vi "tefejaso def3.vi"() -> ()   [LabVIEW 2011]
panel:
  in  "show event/index":bool
  in  "Timeout UDP READ  ms":i32=548
  out "Receive Buffer Size":u32=548
  in  "activetimeout":bool
  out "Active Time Out":bool
  out "Buffer size":u32=548
  in  "Change UDP Parameters":bool
  out "Event Hex":string
  in  "show udp index":bool
  in  "see supertime sec":bool
  in  "see supertime  ns":bool
  in  "see channel":bool
  in  "see tot":bool
  in  "Show channel table":bool
  out "Num Pack 2":u32=1
  out "Supertime ns":u32=1
  out "Supertime sec":u32=1
  out "error time order":bool
  out "error channel":bool
  out "Num Pack":u32=1
  out "Veces canal":u32[](array[numeric])
  out "Table":string[][](table)
  out "num canal":i32=548
  out "Canal TDC":u32[](array[numeric])
  in  "desviacion tipica ancho":dbl
  in  "suma desviacon":dbl
  out "media pulso":dbl
  in  "suma ancho pulso":u32=1
  out "iteracion":i32
  in  "stop":bool
  out "error timestamp":bool
  out "ToT":dynamicdata(graph) caption="Histogram"
  out "Events/TDC channel":dynamicdata(graph) caption="Histogram"
  out "ToT":u32=1
  out "Arrival Time":u32=1
  out "Channel TDC":u32=1
  out "bufferfull":timestamp
  out "UDP INDEX":dynamicdata(graph) caption="Histogram"
  out "EVENT/index":dynamicdata(graph) caption="Histogram"
  out "indice":u32=1
  out "Supertime sec":dynamicdata(graph)
  out "supertime ns":dynamicdata(graph)
  out "current_HRV":u32=1
  out "current_fifo_afull":u32=1
  out "FIFO_FULL":bool[](array[boolean])
  out "HRV":bool[](array[boolean])
  out "Size Packet Bytes":i32
  out "Data Received":string
  in  "max bytes/read":i32=548
  in  "index":u32=1
  out "Port":u16=61557
  out "Num Event":u32=1
  out "START TIME":timestamp
  out "hold_fifo_afull":u32=1
  out "hold_HRV":u32=1
  in  "event/ts":u32=1
  in  "pak_loss":u32=1 caption="packet losses"
  in  "TS_Ch_1":u32=1
  in  "TS_Ch 2":u32=1
  in  "TS_Ch 3":u32=1
  in  "TS_Ch 4":u32=1
  in  "TS_Ch 5":u32=1
  in  "TS_Ch 6":u32=1
  in  "TS_Ch 7":u32=1
  in  "TS_Ch 8":u32=1
  in  "TS_Ch 9":u32=1
  in  "TS_Ch 10":u32=1
  in  "TS_Ch_0":u32=1
  in  "TS_Ch_13":u32=1
  in  "TS_Ch 12":u32=1
  in  "TS_Ch_14":u32=1
  in  "TS_Ch_11":u32=1
  in  "TS_Ch_15":u32=1
  in  "TS_Ch_16":u32=1
  in  "TS_Ch_18":u32=1
  in  "TS_Ch 19":u32=1
  in  "TS_Ch_20":u32=1
  in  "TS_Ch_17":u32=1
  in  "TS_Ch_21":u32=1
  in  "TS_Ch_22":u32=1
  in  "TS_Ch_24":u32=1
  in  "TS_Ch 25":u32=1
  in  "TS_Ch_26":u32=1
  in  "TS_Ch_23":u32=1
  in  "TS_Ch_27":u32=1
  in  "TS_Ch_28":u32=1
  in  "TS_Ch_29":u32=1
  in  "TS_Ch_30":u32=1
  # "TDC DATA MONITOR"
  # "UDP TRANSFER CONDITIONS"
  # "TRANSFER ERRORS"
  # "PACKET INFORMATION"
  # "EVENT INFORMATION"
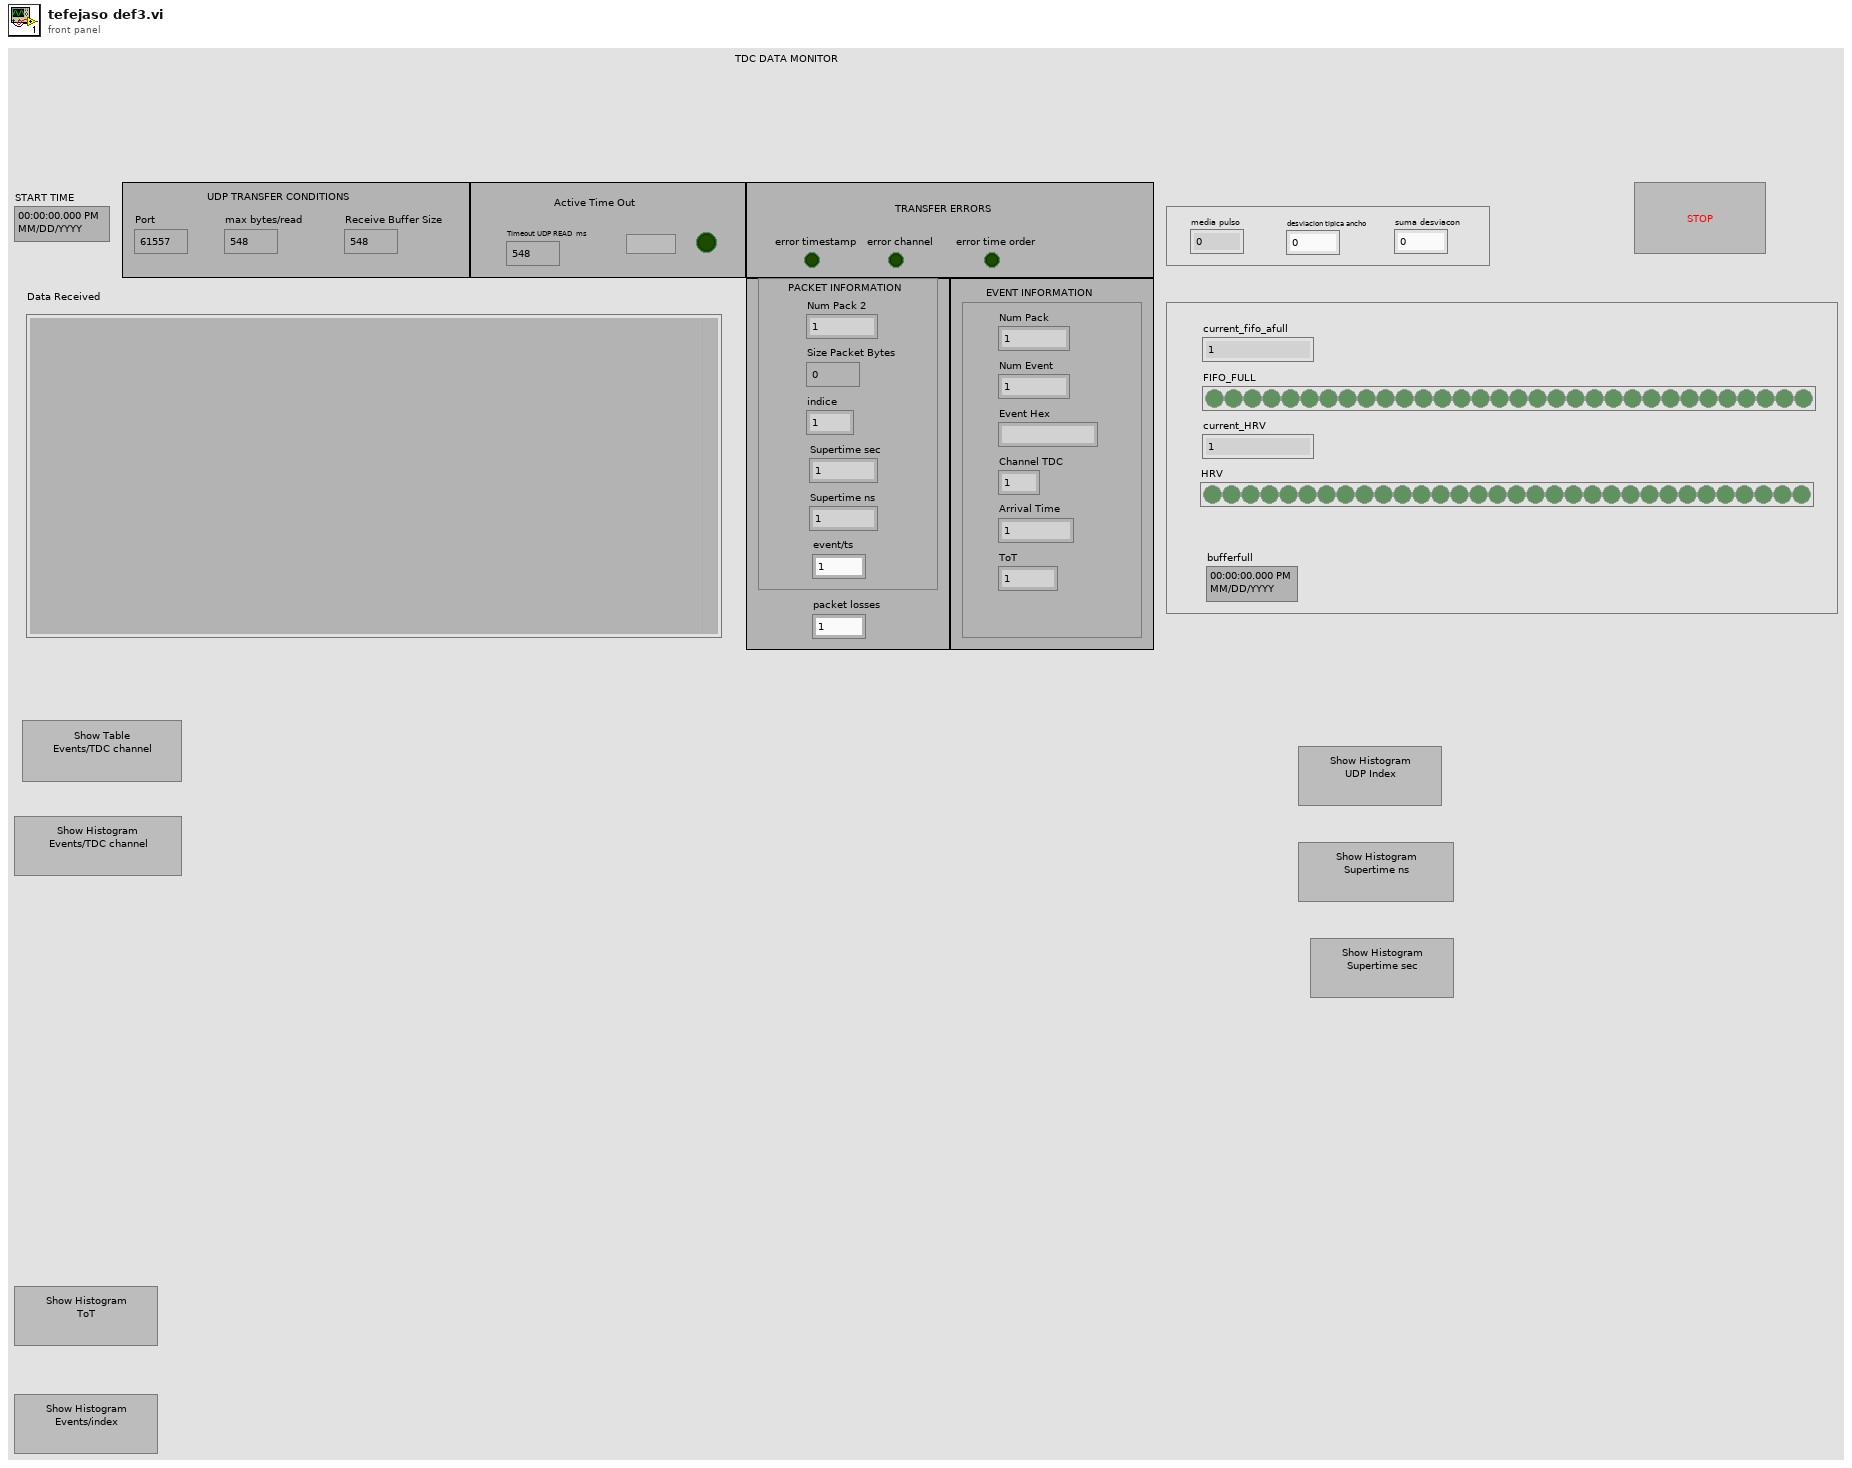
[diagram p1: front panel]
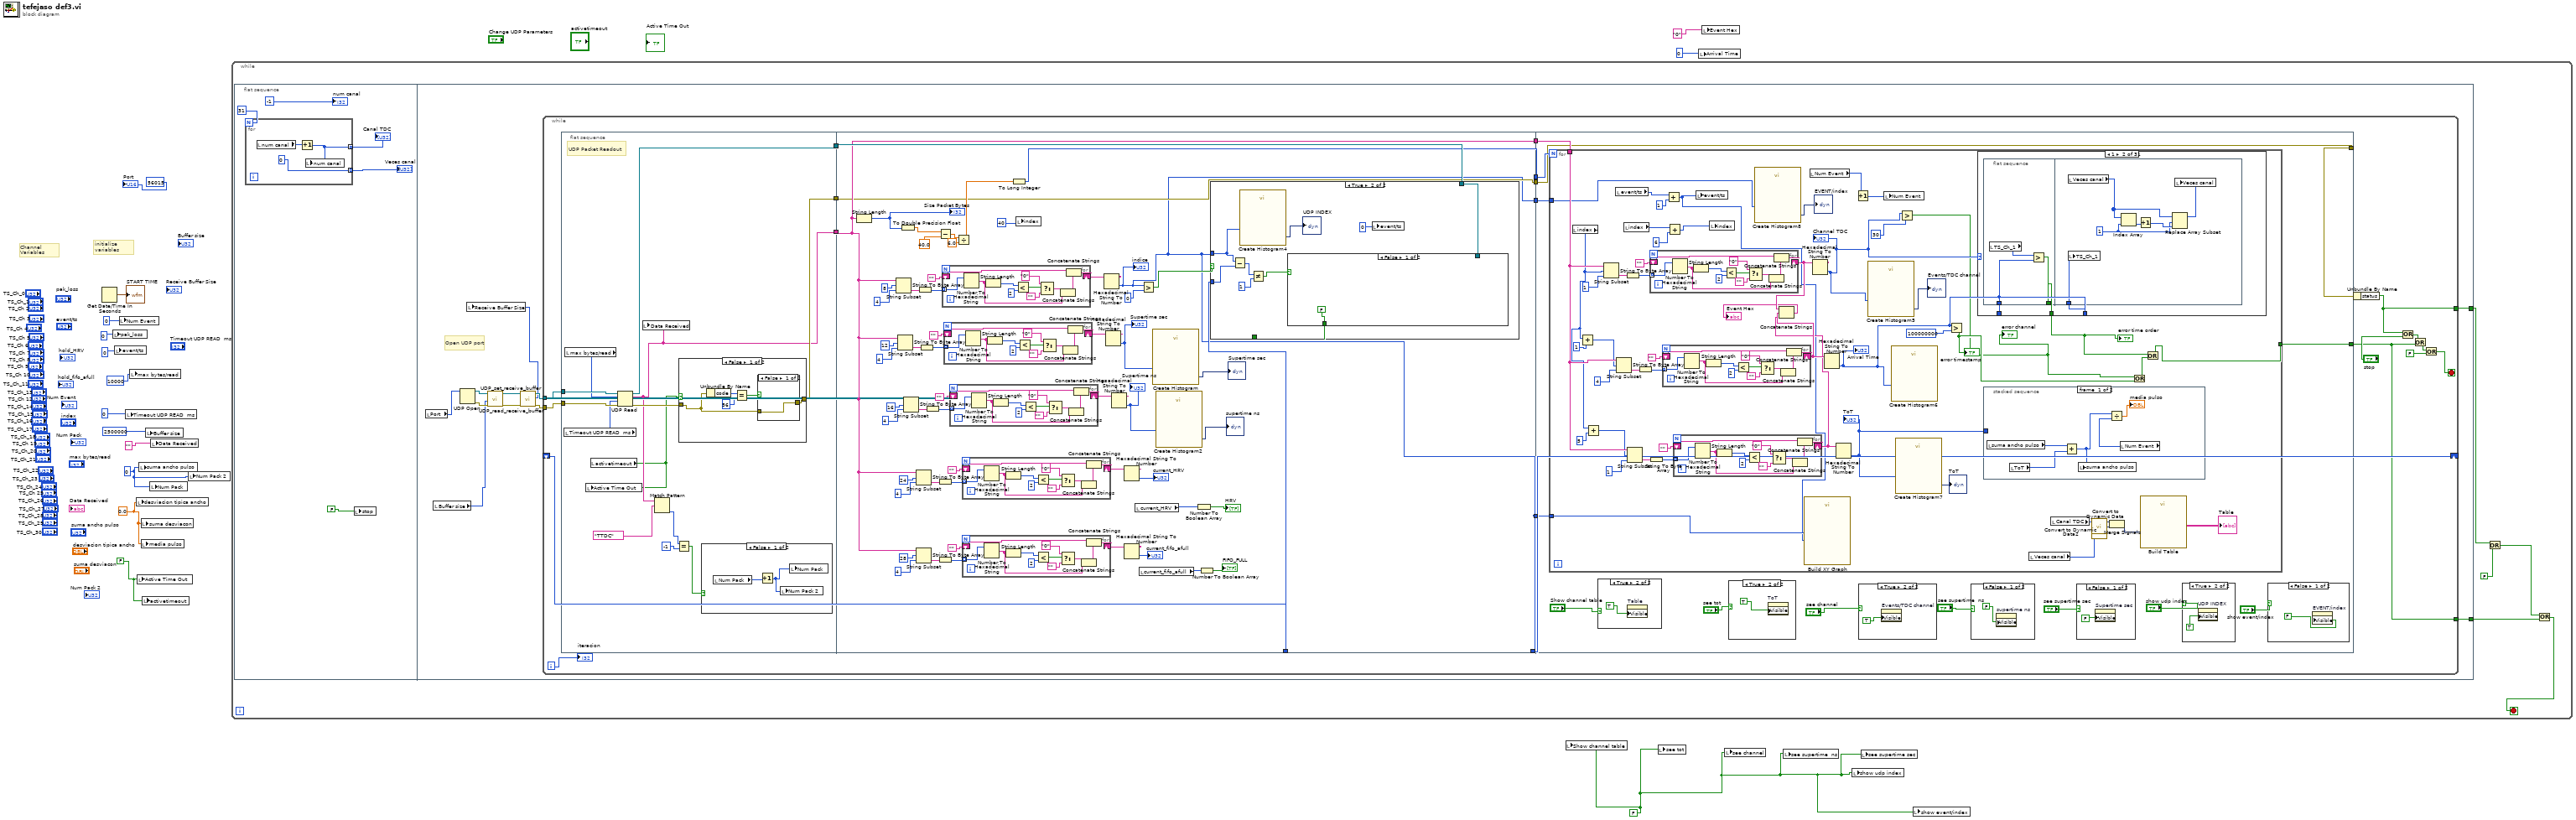
[diagram p0: block diagram]
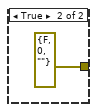
[diagram p2: hidden frame]
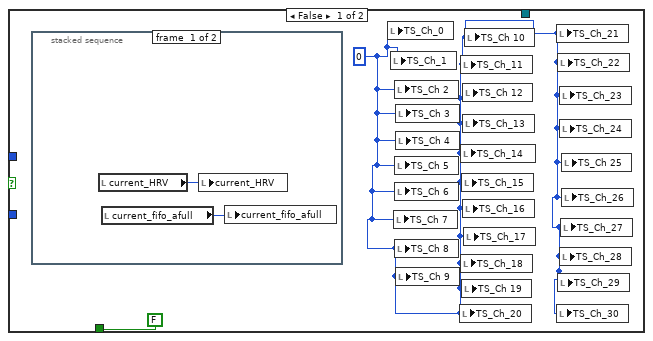
[diagram p5: hidden frame]
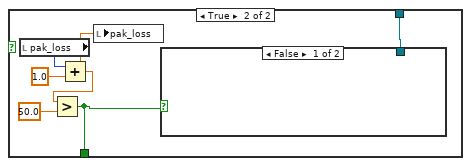
[diagram p7: hidden frame]
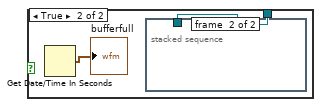
[diagram p8: hidden frame]
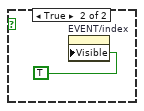
[diagram p10: hidden frame]
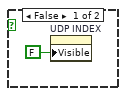
[diagram p11: hidden frame]
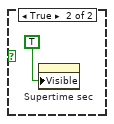
[diagram p12: hidden frame]
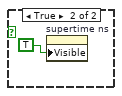
[diagram p13: hidden frame]
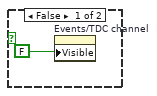
[diagram p14: hidden frame]
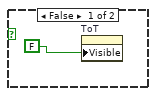
[diagram p15: hidden frame]
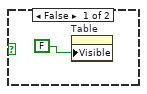
[diagram p16: hidden frame]
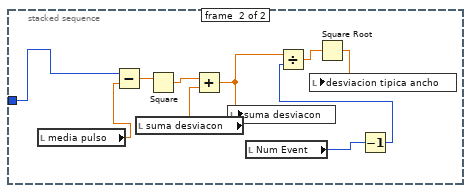
[diagram p17: hidden frame]
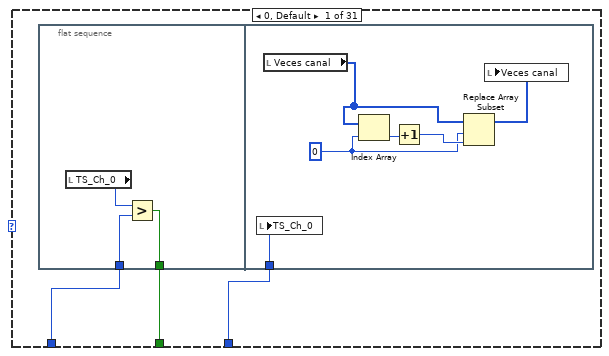
[diagram p18: hidden frame]
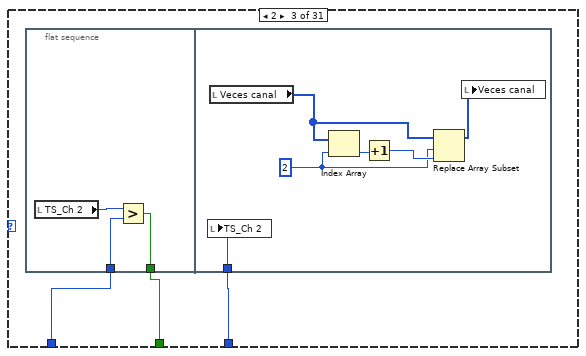
[diagram p19: hidden frame]
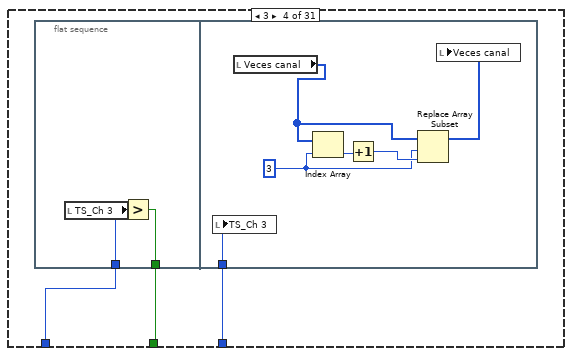
[diagram p20: hidden frame]
diagram:
  w1 = FALSE
  w5 = FALSE
  w9 = 0.0
  w8 = u32 0 ("event/ts")
  # "initialize variables"
  # "Channel Variables"
  n1 = Get Date/Time In Seconds() -> (seconds since 1Jan1904=→"START TIME":timestamp)
  n2 = local write "pak_loss"(u32 0 ("pak_loss")) -> ()
  n3 = local write "event/ts"(u32 0 ("event/ts")) -> ()
  n4 = local write "Num Event"(u32 0 ("contador eventos")) -> ()
  n5 = local write "Timeout UDP READ  ms"(0 ("event/ts")) -> ()
  n6 = local write "max bytes/read"(10000) -> ()
  n7 = local write "desviacion tipica ancho"(w9) -> ()
  n8 = local write "Active Time Out"(w5) -> ()
  n9 = local write "suma ancho pulso"(w8) -> ()
  n10 = local write "suma desviacon"(w9) -> ()
  n11 = local write "media pulso"(w9) -> ()
  n12 = local write "activetimeout"(w5) -> ()
  n13 = local write "Buffer size"(u32 2500000 ("Receive Buffer Size")) -> ()
  n14 = local write "Num Pack"(w8) -> ()
  n15 = local write "Data Received"("") -> ()
  n16 = local write "Num Pack 2"(w8) -> ()
  n17 = while {
    stop <- w17 stop-if-true
    n18 = flat-sequence {
      tunnel: [w33] -> w20
      tunnel: [w29] -> w18
      frame #0 {
        n19 = for {
          N: 31 ("contador eventos") -> [_]
          tunnel: [w27] -> w24 mode=indexing
          tunnel: [u32 0 ("contador eventos")] -> w25 mode=indexing
          n20 = local read "num canal"() -> (w28:i32)
          n21 = Increment(x=w28) -> (x+1=w27:i32)
          n22 = local write "num canal"(w27) -> ()
        }
        "Canal TDC" <- w24
        "Veces canal" <- w25
        n23 = local write "stop"(FALSE) -> ()
        "num canal" <- -1 ("contador eventos")
      }
      frame #1 {
        # "Open UDP port"
        n24 = local read "Port"() -> (w30:u16)
        n25 = local read "Buffer size"() -> (w32:u32)
        n26 = UDP Open(11:w30) -> (port=w36:refnum<k16>, 0:w37:errorcluster)  [unwired: 1 in, 4 out]
        n27 = call "UDP_set_receive_buffer.vi"("error in (no error)"=w37, "Receive Buffer Size"=w32, "connection ID"=w36) -> ("error out"=w39:errorcluster, "connection ID out"=w38:refnum<k16>)  [unwired: 6 in]
        n28 = call "UDP_read_receive_buffer.vi"("error in (no error)"=w39, "connection ID"=w38) -> ("error out"=w34:errorcluster, "Receive Buffer Size"=w31:u32, "connection ID out"=w35:refnum<k16>)  [unwired: 5 in]
        n29 = local write "Receive Buffer Size"(w31) -> ()
        n30 = while {
          tunnel: w35 -> [w60]
          tunnel: w34 -> [w59]
          shift-right: [w44] -> _
          shift-left: _ -> [w45]
          tunnel: [w43] -> w33
          tunnel: [w42] -> w29
          i -> [w46]
          stop <- w49 stop-if-true
          n31 = flat-sequence {
            tunnel: w60 -> [w73]
            tunnel: w59 -> [w72]
            tunnel: [w68] -> w58
            tunnel: [w66] -> w57
            tunnel: [w67] -> w56
            tunnel: w58 -> [w88]
            tunnel: w57 -> [w89]
            tunnel: w56 -> [w93]
            tunnel: [w90] -> w55
            tunnel: [w89] -> w54
            tunnel: [w88] -> w48
            tunnel: w45 -> [w87]
            tunnel: [w84] -> w44
            tunnel: [w84] -> w41
            tunnel: [w84] -> w40
            tunnel: w55 -> [w228]
            tunnel: w54 -> [w227]
            tunnel: [w226] -> w42
            tunnel: [w225] -> w47
            tunnel: w48 -> [w225]
            tunnel: w41 -> [w218]
            tunnel: w40 -> [w217]
            frame #0 {
              # "UDP Packet Readout"
              n32 = local read "Timeout UDP READ  ms"() -> (w70:i32)
              n33 = local read "max bytes/read"() -> (w71:i32)
              n34 = local read "activetimeout"() -> (w61:bool)
              n35 = local write "Active Time Out"(w61) -> ()
              n36 = UDP Read(connection ID=w73, max size (548)=w71, timeout ms (25000)=w70, 8:w72) -> (data out=w66:string, error out=w69:errorcluster, 3:w67:refnum<k16>)  [unwired: 2 out]
              n37 = local write "Data Received"(w66) -> ()
              n38 = Match Pattern(string=w66, regular expression="TTDC") -> (offset past match=w63:i32)  [unwired: 1 in, 3 out]
              n39 = Equal?(x=w63, y=-1) -> (x = y?=w62:bool)
              n40 = case shown="False" w61 {
                tunnel: w69 -> [w75 w81]
                tunnel: [w74 w81] -> w68
                frame False {
                  n41 = Unbundle By Name(w75) -> ("code"=w76:i32)
                  n42 = Equal?(x=w76, y=56) -> (x = y?=w78:bool)
                  n43 = case shown="False" w78 {
                    tunnel: w75 -> [w79 _]
                    tunnel: [w79 errorcluster {"status"=FALSE, "code"=0, "source"=""} ("error out")] -> w74
                    frame False {
                    }
                    frame True {
                    }
                  }
                }
                frame True {
                }
              }
              n44 = case shown="False" w62 {
                frame False {
                  n45 = local read "Num Pack"() -> (w82:u32)
                  n46 = Increment(x=w82) -> (x+1=w83:u32)
                  n47 = local write "Num Pack 2"(w83) -> ()
                  n48 = local write "Num Pack"(w83) -> ()
                }
                frame True {
                }
              }
            }
            frame #1 {
              n49 = String Length(string=w89) -> (length=w105:i32)
              "Size Packet Bytes" <- w105
              n50 = String Subset(string=w89, offset (0)=8, length (rest)=4) -> (substring=w135:string)
              n51 = String Subset(string=w89, offset (0)=12, length (rest)=4) -> (substring=w129:string)
              n52 = To Double Precision Float(number=w105) -> (double precision float=w104:dbl)
              n53 = String Subset(string=w89, offset (0)=16, length (rest)=4) -> (substring=w123:string)
              n54 = String Subset(string=w89, offset (0)=24, length (rest)=4) -> (substring=w117:string)
              n55 = String Subset(string=w89, offset (0)=28, length (rest)=4) -> (substring=w111:string)
              n56 = String To Byte Array(string=w135) -> (unsigned byte array=w133:u8[])
              n57 = String To Byte Array(string=w129) -> (unsigned byte array=w127:u8[])
              n58 = String To Byte Array(string=w123) -> (unsigned byte array=w121:u8[])
              n59 = String To Byte Array(string=w117) -> (unsigned byte array=w115:u8[])
              n60 = String To Byte Array(string=w111) -> (unsigned byte array=w109:u8[])
              n61 = Subtract(x=w104, y=40.0) -> (x-y=w108:dbl)
              n62 = for {
                tunnel: w133 -> [w205] mode=indexing
                shift-right: [w206] -> w137
                shift-left: "" -> [w207]
                n63 = Number To Hexadecimal String(2:w205) -> (0:w209:string)  [unwired: 1 in]
                n64 = String Length(string=w209) -> (length=w215:i32)
                n65 = Less?(x=w215, y=2) -> (x < y?=w212:bool)
                n66 = Select(t="0", s=w212, f="") -> (s? t:f=w210:string)
                n67 = Concatenate Strings(w210, w209) -> (w208:string)
                n68 = Concatenate Strings(w207, w208) -> (w206:string)
              }
              n69 = for {
                tunnel: w127 -> [w194] mode=indexing
                shift-right: [w195] -> w131
                shift-left: "" -> [w196]
                n70 = Number To Hexadecimal String(2:w194) -> (0:w198:string)  [unwired: 1 in]
                n71 = String Length(string=w198) -> (length=w204:i32)
                n72 = Less?(x=w204, y=2) -> (x < y?=w201:bool)
                n73 = Select(t="0", s=w201, f="") -> (s? t:f=w199:string)
                n74 = Concatenate Strings(w199, w198) -> (w197:string)
                n75 = Concatenate Strings(w196, w197) -> (w195:string)
              }
              n76 = for {
                tunnel: w121 -> [w183] mode=indexing
                shift-right: [w184] -> w125
                shift-left: "" -> [w185]
                n77 = Number To Hexadecimal String(2:w183) -> (0:w187:string)  [unwired: 1 in]
                n78 = String Length(string=w187) -> (length=w193:i32)
                n79 = Less?(x=w193, y=2) -> (x < y?=w190:bool)
                n80 = Select(t="0", s=w190, f="") -> (s? t:f=w188:string)
                n81 = Concatenate Strings(w188, w187) -> (w186:string)
                n82 = Concatenate Strings(w185, w186) -> (w184:string)
              }
              n83 = Divide(x=w108, y=6.0) -> (x/y=w91:dbl)
              n84 = for {
                tunnel: w115 -> [w172] mode=indexing
                shift-right: [w173] -> w119
                shift-left: "" -> [w174]
                n85 = Number To Hexadecimal String(2:w172) -> (0:w176:string)  [unwired: 1 in]
                n86 = String Length(string=w176) -> (length=w182:i32)
                n87 = Less?(x=w182, y=2) -> (x < y?=w179:bool)
                n88 = Select(t="0", s=w179, f="") -> (s? t:f=w177:string)
                n89 = Concatenate Strings(w177, w176) -> (w175:string)
                n90 = Concatenate Strings(w174, w175) -> (w173:string)
              }
              n91 = for {
                tunnel: w109 -> [w161] mode=indexing
                shift-right: [w162] -> w113
                shift-left: "" -> [w163]
                n92 = Number To Hexadecimal String(2:w161) -> (0:w165:string)  [unwired: 1 in]
                n93 = String Length(string=w165) -> (length=w171:i32)
                n94 = Less?(x=w171, y=2) -> (x < y?=w168:bool)
                n95 = Select(t="0", s=w168, f="") -> (s? t:f=w166:string)
                n96 = Concatenate Strings(w166, w165) -> (w164:string)
                n97 = Concatenate Strings(w163, w164) -> (w162:string)
              }
              n98 = To Long Integer(number=w91) -> (32bit integer=w90:i32)
              n99 = local write "index"(u32 40 ("index")) -> ()
              n100 = Hexadecimal String To Number(string=w137) -> (number=w84:u32)  [unwired: 2 in, 1 out]
              "indice" <- w84
              n101 = Hexadecimal String To Number(string=w131) -> (number=w86:u32)  [unwired: 2 in, 1 out]
              "Supertime sec" <- w86
              n102 = Hexadecimal String To Number(string=w125) -> (number=w85:u32)  [unwired: 2 in, 1 out]
              "Supertime ns" <- w85
              n103 = Hexadecimal String To Number(string=w119) -> (number=→"current_HRV":u32)  [unwired: 2 in, 1 out]
              n104 = Hexadecimal String To Number(string=w113) -> (number=→"current_fifo_afull":u32)  [unwired: 2 in, 1 out]
              n105 = local read "current_HRV"() -> (w96:u32)
              n106 = local read "current_fifo_afull"() -> (w95:u32)
              n107 = Greater?(x=w84, y=u32 0 ("index")) -> (0:w92:bool)
              n108 = call "Create Histogram"("Signal"=w86) -> ("Histogram"=→"Supertime sec":dynamicdata)  [unwired: 9 in, 1 out]
              n109 = call "Create Histogram2"("Signal"=w85) -> ("Histogram"=→"supertime ns":dynamicdata)  [unwired: 9 in, 1 out]
              n110 = Number To Boolean Array(number=w96) -> (Boolean array=→"HRV":bool[])
              n111 = Number To Boolean Array(number=w95) -> (Boolean array=→"FIFO_FULL":bool[])
              n112 = case shown="True" w92 {
                tunnel: w84 -> [_ w145]
                tunnel: w87 -> [_ w151]
                tunnel: [FALSE w148] -> _
                tunnel: w93 -> [_ w147]
                frame False {
                  w139 = u32 0 ("TS_Ch 10")
                  n113 = stacked-sequence {
                    frame #0 {
                      n114 = local read "current_HRV"() -> (w142:u32)
                      n115 = local read "current_fifo_afull"() -> (w141:u32)
                      n116 = local write "current_HRV"(w142) -> ()
                      n117 = local write "current_fifo_afull"(w141) -> ()
                    }
                    frame #1 {
                    }
                  }
                  n118 = local write "TS_Ch_0"(w139) -> ()
                  n119 = local write "TS_Ch_1"(w139) -> ()
                  n120 = local write "TS_Ch 7"(w139) -> ()
                  n121 = local write "TS_Ch 2"(w139) -> ()
                  n122 = local write "TS_Ch 5"(w139) -> ()
                  n123 = local write "TS_Ch 6"(w139) -> ()
                  n124 = local write "TS_Ch 8"(w139) -> ()
                  n125 = local write "TS_Ch 3"(w139) -> ()
                  n126 = local write "TS_Ch 4"(w139) -> ()
                  n127 = local write "TS_Ch 9"(w139) -> ()
                  n128 = local write "TS_Ch_20"(w139) -> ()
                  n129 = local write "TS_Ch_11"(w139) -> ()
                  n130 = local write "TS_Ch_14"(w139) -> ()
                  n131 = local write "TS_Ch_18"(w139) -> ()
                  n132 = local write "TS_Ch_15"(w139) -> ()
                  n133 = local write "TS_Ch 19"(w139) -> ()
                  n134 = local write "TS_Ch 12"(w139) -> ()
                  n135 = local write "TS_Ch_13"(w139) -> ()
                  n136 = local write "TS_Ch_16"(w139) -> ()
                  n137 = local write "TS_Ch_17"(w139) -> ()
                  n138 = local write "TS_Ch 10"(w139) -> ()
                  n139 = local write "TS_Ch_21"(w139) -> ()
                  n140 = local write "TS_Ch_30"(w139) -> ()
                  n141 = local write "TS_Ch_22"(w139) -> ()
                  n142 = local write "TS_Ch_29"(w139) -> ()
                  n143 = local write "TS_Ch_23"(w139) -> ()
                  n144 = local write "TS_Ch_24"(w139) -> ()
                  n145 = local write "TS_Ch_28"(w139) -> ()
                  n146 = local write "TS_Ch_27"(w139) -> ()
                  n147 = local write "TS_Ch 25"(w139) -> ()
                  n148 = local write "TS_Ch_26"(w139) -> ()
                }
                frame True {
                  n149 = Subtract(x=w145, y=w151) -> (x-y=w150:u32)
                  n150 = call "Create Histogram4"("Signal"=w145) -> ("Histogram"=→"UDP INDEX":dynamicdata)  [unwired: 9 in, 1 out]
                  n151 = Not Equal?(x=w150, y=u32 1) -> (x != y?=w144:bool)
                  n152 = case shown="False" w144 {
                    tunnel: [FALSE w154] -> w148
                    tunnel: w147 -> [_ w153]
                    frame False {
                    }
                    frame True {
                      n153 = local read "pak_loss"() -> (w158:u32)
                      n154 = Add(x=w158, y=1.0) -> (x+y=w155:dbl)
                      n155 = Greater?(x=w155, y=50.0) -> (0:w154:bool)
                      n156 = local write "pak_loss"(w155) -> ()
                      n157 = case shown="False" w154 {
                        tunnel: w153 -> [_ w159]
                        frame False {
                        }
                        frame True {
                          n158 = Get Date/Time In Seconds() -> (seconds since 1Jan1904=→"bufferfull":timestamp)
                          n159 = stacked-sequence {
                            tunnel: w159 -> [_ _]
                            frame #0 {
                            }
                            frame #1 {
                            }
                          }
                        }
                      }
                    }
                  }
                  n160 = local write "event/ts"(u32 0 ("event/ts")) -> ()
                }
              }
            }
            frame #2 {
              n161 = for {
                N: w228 -> [_]
                tunnel: w227 -> [w281]
                tunnel: [w268] -> w226
                tunnel: w218 -> [w245]
                tunnel: w217 -> [w244]
                n162 = local read "index"() -> (w262:u32)
                n163 = Add(x=w262, y=u32 1) -> (x+y=w265:u32)
                n164 = Add(x=w262, y=u32 5 ("offset (0)")) -> (x+y=w264:u32)
                n165 = String Subset(string=w281, offset (0)=w262, length (rest)=1) -> (substring=w292:string)
                n166 = local read "event/ts"() -> (w280:u32)
                n167 = String Subset(string=w281, offset (0)=w265, length (rest)=4) -> (substring=w288:string)
                n168 = local read "index"() -> (w267:u32)
                n169 = String To Byte Array(string=w292) -> (unsigned byte array=w290:u8[])
                n170 = String Subset(string=w281, offset (0)=w264, length (rest)=1) -> (substring=w284:string)
                n171 = String To Byte Array(string=w288) -> (unsigned byte array=w286:u8[])
                n172 = String To Byte Array(string=w284) -> (unsigned byte array=w282:u8[])
                n173 = for {
                  tunnel: w290 -> [w703] mode=indexing
                  shift-right: [w704] -> w250
                  shift-left: "" -> [w705]
                  n174 = Number To Hexadecimal String(2:w703) -> (0:w707:string)  [unwired: 1 in]
                  n175 = String Length(string=w707) -> (length=w713:i32)
                  n176 = Less?(x=w713, y=2) -> (x < y?=w710:bool)
                  n177 = Select(t="0", s=w710, f="") -> (s? t:f=w708:string)
                  n178 = Concatenate Strings(w708, w707) -> (w706:string)
                  n179 = Concatenate Strings(w705, w706) -> (w704:string)
                }
                n180 = for {
                  tunnel: w286 -> [w692] mode=indexing
                  shift-right: [w693] -> w249
                  shift-left: "" -> [w694]
                  n181 = Number To Hexadecimal String(2:w692) -> (0:w696:string)  [unwired: 1 in]
                  n182 = String Length(string=w696) -> (length=w702:i32)
                  n183 = Less?(x=w702, y=2) -> (x < y?=w699:bool)
                  n184 = Select(t="0", s=w699, f="") -> (s? t:f=w697:string)
                  n185 = Concatenate Strings(w697, w696) -> (w695:string)
                  n186 = Concatenate Strings(w694, w695) -> (w693:string)
                }
                n187 = Add(x=w280, y=u32 1) -> (x+y=w243:u32)
                n188 = Add(x=w267, y=u32 6) -> (x+y=w277:u32)
                n189 = for {
                  tunnel: w282 -> [w681] mode=indexing
                  shift-right: [w682] -> w248
                  shift-left: "" -> [w683]
                  n190 = Number To Hexadecimal String(2:w681) -> (0:w685:string)  [unwired: 1 in]
                  n191 = String Length(string=w685) -> (length=w691:i32)
                  n192 = Less?(x=w691, y=2) -> (x < y?=w688:bool)
                  n193 = Select(t="0", s=w688, f="") -> (s? t:f=w686:string)
                  n194 = Concatenate Strings(w686, w685) -> (w684:string)
                  n195 = Concatenate Strings(w683, w684) -> (w682:string)
                }
                n196 = local write "event/ts"(w243) -> ()
                n197 = local write "index"(w277) -> ()
                n198 = call "Create Histogram8"("Signal"=w244) -> ("Histogram"=→"EVENT/index":dynamicdata)  [unwired: 9 in, 1 out]
                n199 = Concatenate Strings(w250, w249, w248) -> (→"Event Hex":string)
                n200 = call "Build XY Graph"("Y Input"=w243, "X Input"=w245) -> ()  [unwired: 3 in, 7 out]
                n201 = local read "Num Event"() -> (w273:u32)
                n202 = Hexadecimal String To Number(string=w250) -> (number=w256:u32)  [unwired: 2 in, 1 out]
                "Channel TDC" <- w256
                n203 = Hexadecimal String To Number(string=w249) -> (number=w269:u32)  [unwired: 2 in, 1 out]
                "Arrival Time" <- w269
                n204 = Hexadecimal String To Number(string=w248) -> (number=w260:u32)  [unwired: 2 in, 1 out]
                "ToT" <- w260
                n205 = Increment(x=w273) -> (x+1=w272:u32)
                n206 = call "Create Histogram5"("Signal"=w256) -> ("Histogram"=→"Events/TDC channel":dynamicdata)  [unwired: 9 in, 1 out]
                n207 = local write "Num Event"(w272) -> ()
                n208 = call "Create Histogram6"("Signal"=w269) -> ()  [unwired: 9 in, 2 out]
                n209 = call "Create Histogram7"("Signal"=w260) -> ("Histogram"=→"ToT":dynamicdata)  [unwired: 9 in, 1 out]
                n210 = Greater?(x=w256, y=u32 30) -> (0:w252:bool)
                "error channel" <- w252
                n211 = Greater?(x=w269, y=u32 100000000 ("x")) -> (0:w271:bool)
                "error timestamp" <- w271
                n212 = case shown="1" w256 {
                  tunnel: w269 -> [w310 w323 w334 w346 w358 w370 w382 w394 w406 w418 w430 w442 w454 w466 w478 w490 w502 w514 w526 w538 w550 w562 w574 w586 w598 w610 w622 w634 w646 w658 w671]
                  tunnel: w269 -> [w311 w322 w335 w347 w359 w371 w383 w395 w407 w419 w431 w443 w455 w467 w479 w491 w503 w515 w527 w539 w551 w563 w575 w587 w599 w611 w623 w635 w647 w659 w670]
                  tunnel: [w309 w321 w333 w345 w357 w369 w381 w393 w405 w417 w429 w441 w453 w465 w477 w489 w501 w513 w525 w537 w549 w561 w573 w585 w597 w609 w621 w633 w645 w657 w669] -> w251
                  frame 0, Default {
                    n213 = flat-sequence {
                      tunnel: w311 -> [w313]
                      tunnel: [w312] -> w309
                      tunnel: w310 -> [w320]
                      frame #0 {
                        n214 = local read "TS_Ch_0"() -> (w314:u32)
                        n215 = Greater?(x=w314, y=w313) -> (0:w312:bool)
                      }
                      frame #1 {
                        w317 = 0 ("contador eventos")
                        n216 = local write "TS_Ch_0"(w320) -> ()
                        n217 = local read "Veces canal"() -> (w316:u32[])
                        n218 = Index Array(array=w316, index=w317) -> (element=w318:u32)
                        n219 = Increment(x=w318) -> (x+1=w319:u32)
                        n220 = Replace Array Subset(array=w316, new element=w319, index=w317) -> (w315:u32[])
                        n221 = local write "Veces canal"(w315) -> ()
                      }
                    }
                  }
                  frame 1 {
                    n222 = flat-sequence {
                      tunnel: w322 -> [w326]
                      tunnel: [w324] -> w321
                      tunnel: w323 -> [w332]
                      frame #0 {
                        n223 = local read "TS_Ch_1"() -> (w325:u32)
                        n224 = Greater?(x=w325, y=w326) -> (0:w324:bool)
                      }
                      frame #1 {
                        w329 = 1 ("contador eventos")
                        n225 = local read "Veces canal"() -> (w328:u32[])
                        n226 = local write "TS_Ch_1"(w332) -> ()
                        n227 = Index Array(array=w328, index=w329) -> (element=w330:u32)
                        n228 = Increment(x=w330) -> (x+1=w331:u32)
                        n229 = Replace Array Subset(array=w328, new element=w331, index=w329) -> (w327:u32[])
                        n230 = local write "Veces canal"(w327) -> ()
                      }
                    }
                  }
                  frame 2 {
                    n231 = flat-sequence {
                      tunnel: w335 -> [w337]
                      tunnel: [w336] -> w333
                      tunnel: w334 -> [w344]
                      frame #0 {
                        n232 = local read "TS_Ch 2"() -> (w338:u32)
                        n233 = Greater?(x=w338, y=w337) -> (0:w336:bool)
                      }
                      frame #1 {
                        w339 = 2 ("contador eventos")
                        n234 = local write "TS_Ch 2"(w344) -> ()
                        n235 = local read "Veces canal"() -> (w342:u32[])
                        n236 = Index Array(array=w342, index=w339) -> (element=w340:u32)
                        n237 = Increment(x=w340) -> (x+1=w341:u32)
                        n238 = Replace Array Subset(array=w342, new element=w341, index=w339) -> (w343:u32[])
                        n239 = local write "Veces canal"(w343) -> ()
                      }
                    }
                  }
                  frame 3 {
                    n240 = flat-sequence {
                      tunnel: w347 -> [w349]
                      tunnel: [w348] -> w345
                      tunnel: w346 -> [w356]
                      frame #0 {
                        n241 = local read "TS_Ch 3"() -> (w350:u32)
                        n242 = Greater?(x=w350, y=w349) -> (0:w348:bool)
                      }
                      frame #1 {
                        w353 = 3 ("contador eventos")
                        n243 = local write "TS_Ch 3"(w356) -> ()
                        n244 = local read "Veces canal"() -> (w352:u32[])
                        n245 = Index Array(array=w352, index=w353) -> (element=w354:u32)
                        n246 = Increment(x=w354) -> (x+1=w355:u32)
                        n247 = Replace Array Subset(array=w352, new element=w355, index=w353) -> (w351:u32[])
                        n248 = local write "Veces canal"(w351) -> ()
                      }
                    }
                  }
                  frame 4 {
                    n249 = flat-sequence {
                      tunnel: w359 -> [w361]
                      tunnel: [w360] -> w357
                      tunnel: w358 -> [w368]
                      frame #0 {
                        n250 = local read "TS_Ch 4"() -> (w362:u32)
                        n251 = Greater?(x=w362, y=w361) -> (0:w360:bool)
                      }
                      frame #1 {
                        w365 = 4 ("contador eventos")
                        n252 = local write "TS_Ch 4"(w368) -> ()
                        n253 = local read "Veces canal"() -> (w364:u32[])
                        n254 = Index Array(array=w364, index=w365) -> (element=w366:u32)
                        n255 = Increment(x=w366) -> (x+1=w367:u32)
                        n256 = Replace Array Subset(array=w364, new element=w367, index=w365) -> (w363:u32[])
                        n257 = local write "Veces canal"(w363) -> ()
                      }
                    }
                  }
                  frame 5 {
                    n258 = flat-sequence {
                      tunnel: w371 -> [w373]
                      tunnel: [w372] -> w369
                      tunnel: w370 -> [w380]
                      frame #0 {
                        n259 = local read "TS_Ch 5"() -> (w374:u32)
                        n260 = Greater?(x=w374, y=w373) -> (0:w372:bool)
                      }
                      frame #1 {
                        w377 = 5 ("contador eventos")
                        n261 = local write "TS_Ch 5"(w380) -> ()
                        n262 = local read "Veces canal"() -> (w376:u32[])
                        n263 = Index Array(array=w376, index=w377) -> (element=w378:u32)
                        n264 = Increment(x=w378) -> (x+1=w379:u32)
                        n265 = Replace Array Subset(array=w376, new element=w379, index=w377) -> (w375:u32[])
                        n266 = local write "Veces canal"(w375) -> ()
                      }
                    }
                  }
                  frame 6 {
                    n267 = flat-sequence {
                      tunnel: w383 -> [w385]
                      tunnel: [w384] -> w381
                      tunnel: w382 -> [w392]
                      frame #0 {
                        n268 = local read "TS_Ch 6"() -> (w386:u32)
                        n269 = Greater?(x=w386, y=w385) -> (0:w384:bool)
                      }
                      frame #1 {
                        w389 = 6 ("contador eventos")
                        n270 = local write "TS_Ch 6"(w392) -> ()
                        n271 = local read "Veces canal"() -> (w388:u32[])
                        n272 = Index Array(array=w388, index=w389) -> (element=w390:u32)
                        n273 = Increment(x=w390) -> (x+1=w391:u32)
                        n274 = Replace Array Subset(array=w388, new element=w391, index=w389) -> (w387:u32[])
                        n275 = local write "Veces canal"(w387) -> ()
                      }
                    }
                  }
                  frame 7 {
                    n276 = flat-sequence {
                      tunnel: w395 -> [w397]
                      tunnel: [w396] -> w393
                      tunnel: w394 -> [w404]
                      frame #0 {
                        n277 = local read "TS_Ch 7"() -> (w398:u32)
                        n278 = Greater?(x=w398, y=w397) -> (0:w396:bool)
                      }
                      frame #1 {
                        w401 = 7 ("contador eventos")
                        n279 = local write "TS_Ch 7"(w404) -> ()
                        n280 = local read "Veces canal"() -> (w400:u32[])
                        n281 = Index Array(array=w400, index=w401) -> (element=w402:u32)
                        n282 = Increment(x=w402) -> (x+1=w403:u32)
                        n283 = Replace Array Subset(array=w400, new element=w403, index=w401) -> (w399:u32[])
                        n284 = local write "Veces canal"(w399) -> ()
                      }
                    }
                  }
                  frame 8 {
                    n285 = flat-sequence {
                      tunnel: w407 -> [w409]
                      tunnel: [w408] -> w405
                      tunnel: w406 -> [w416]
                      frame #0 {
                        n286 = local read "TS_Ch 8"() -> (w410:u32)
                        n287 = Greater?(x=w410, y=w409) -> (0:w408:bool)
                      }
                      frame #1 {
                        w413 = 8 ("contador eventos")
                        n288 = local write "TS_Ch 8"(w416) -> ()
                        n289 = local read "Veces canal"() -> (w412:u32[])
                        n290 = Index Array(array=w412, index=w413) -> (element=w414:u32)
                        n291 = Increment(x=w414) -> (x+1=w415:u32)
                        n292 = Replace Array Subset(array=w412, new element=w415, index=w413) -> (w411:u32[])
                        n293 = local write "Veces canal"(w411) -> ()
                      }
                    }
                  }
                  frame 9 {
                    n294 = flat-sequence {
                      tunnel: w419 -> [w421]
                      tunnel: [w420] -> w417
                      tunnel: w418 -> [w428]
                      frame #0 {
                        n295 = local read "TS_Ch 9"() -> (w422:u32)
                        n296 = Greater?(x=w422, y=w421) -> (0:w420:bool)
                      }
                      frame #1 {
                        w425 = 9 ("contador eventos")
                        n297 = local write "TS_Ch 9"(w428) -> ()
                        n298 = local read "Veces canal"() -> (w424:u32[])
                        n299 = Index Array(array=w424, index=w425) -> (element=w426:u32)
                        n300 = Increment(x=w426) -> (x+1=w427:u32)
                        n301 = Replace Array Subset(array=w424, new element=w427, index=w425) -> (w423:u32[])
                        n302 = local write "Veces canal"(w423) -> ()
                      }
                    }
                  }
                  frame 10 {
                    n303 = flat-sequence {
                      tunnel: w431 -> [w433]
                      tunnel: [w432] -> w429
                      tunnel: w430 -> [w440]
                      frame #0 {
                        n304 = local read "TS_Ch 10"() -> (w434:u32)
                        n305 = Greater?(x=w434, y=w433) -> (0:w432:bool)
                      }
                      frame #1 {
                        w437 = 10 ("contador eventos")
                        n306 = local write "TS_Ch 10"(w440) -> ()
                        n307 = local read "Veces canal"() -> (w436:u32[])
                        n308 = Index Array(array=w436, index=w437) -> (element=w438:u32)
                        n309 = Increment(x=w438) -> (x+1=w439:u32)
                        n310 = Replace Array Subset(array=w436, new element=w439, index=w437) -> (w435:u32[])
                        n311 = local write "Veces canal"(w435) -> ()
                      }
                    }
                  }
                  frame 11 {
                    n312 = flat-sequence {
                      tunnel: w443 -> [w445]
                      tunnel: [w444] -> w441
                      tunnel: w442 -> [w452]
                      frame #0 {
                        n313 = local read "TS_Ch_11"() -> (w446:u32)
                        n314 = Greater?(x=w446, y=w445) -> (0:w444:bool)
                      }
                      frame #1 {
                        w449 = 11 ("contador eventos")
                        n315 = local write "TS_Ch_11"(w452) -> ()
                        n316 = local read "Veces canal"() -> (w447:u32[])
                        n317 = Index Array(array=w447, index=w449) -> (element=w450:u32)
                        n318 = Increment(x=w450) -> (x+1=w451:u32)
                        n319 = Replace Array Subset(array=w447, new element=w451, index=w449) -> (w448:u32[])
                        n320 = local write "Veces canal"(w448) -> ()
                      }
                    }
                  }
                  frame 12 {
                    n321 = flat-sequence {
                      tunnel: w455 -> [w457]
                      tunnel: [w456] -> w453
                      tunnel: w454 -> [w464]
                      frame #0 {
                        n322 = local read "TS_Ch 12"() -> (w458:u32)
                        n323 = Greater?(x=w458, y=w457) -> (0:w456:bool)
                      }
                      frame #1 {
                        w461 = 12 ("contador eventos")
                        n324 = local read "Veces canal"() -> (w459:u32[])
                        n325 = local write "TS_Ch 12"(w464) -> ()
                        n326 = Index Array(array=w459, index=w461) -> (element=w462:u32)
                        n327 = Increment(x=w462) -> (x+1=w463:u32)
                        n328 = Replace Array Subset(array=w459, new element=w463, index=w461) -> (w460:u32[])
                        n329 = local write "Veces canal"(w460) -> ()
                      }
                    }
                  }
                  frame 13 {
                    n330 = flat-sequence {
                      tunnel: w467 -> [w469]
                      tunnel: [w468] -> w465
                      tunnel: w466 -> [w476]
                      frame #0 {
                        n331 = local read "TS_Ch_13"() -> (w470:u32)
                        n332 = Greater?(x=w470, y=w469) -> (0:w468:bool)
                      }
                      frame #1 {
                        w473 = 13 ("contador eventos")
                        n333 = local read "Veces canal"() -> (w471:u32[])
                        n334 = local write "TS_Ch_13"(w476) -> ()
                        n335 = Index Array(array=w471, index=w473) -> (element=w474:u32)
                        n336 = Increment(x=w474) -> (x+1=w475:u32)
                        n337 = Replace Array Subset(array=w471, new element=w475, index=w473) -> (w472:u32[])
                        n338 = local write "Veces canal"(w472) -> ()
                      }
                    }
                  }
                  frame 14 {
                    n339 = flat-sequence {
                      tunnel: w479 -> [w481]
                      tunnel: [w480] -> w477
                      tunnel: w478 -> [w488]
                      frame #0 {
                        n340 = local read "TS_Ch_14"() -> (w482:u32)
                        n341 = Greater?(x=w482, y=w481) -> (0:w480:bool)
                      }
                      frame #1 {
                        w485 = 14 ("contador eventos")
                        n342 = local write "TS_Ch_14"(w488) -> ()
                        n343 = local read "Veces canal"() -> (w483:u32[])
                        n344 = Index Array(array=w483, index=w485) -> (element=w486:u32)
                        n345 = Increment(x=w486) -> (x+1=w487:u32)
                        n346 = Replace Array Subset(array=w483, new element=w487, index=w485) -> (w484:u32[])
                        n347 = local write "Veces canal"(w484) -> ()
                      }
                    }
                  }
                  frame 15 {
                    n348 = flat-sequence {
                      tunnel: w491 -> [w493]
                      tunnel: [w492] -> w489
                      tunnel: w490 -> [w500]
                      frame #0 {
                        n349 = local read "TS_Ch_15"() -> (w494:u32)
                        n350 = Greater?(x=w494, y=w493) -> (0:w492:bool)
                      }
                      frame #1 {
                        w497 = 15 ("contador eventos")
                        n351 = local write "TS_Ch_15"(w500) -> ()
                        n352 = local read "Veces canal"() -> (w495:u32[])
                        n353 = Index Array(array=w495, index=w497) -> (element=w498:u32)
                        n354 = Increment(x=w498) -> (x+1=w499:u32)
                        n355 = Replace Array Subset(array=w495, new element=w499, index=w497) -> (w496:u32[])
                        n356 = local write "Veces canal"(w496) -> ()
                      }
                    }
                  }
                  frame 16 {
                    n357 = flat-sequence {
                      tunnel: w503 -> [w505]
                      tunnel: [w504] -> w501
                      tunnel: w502 -> [w512]
                      frame #0 {
                        n358 = local read "TS_Ch_16"() -> (w506:u32)
                        n359 = Greater?(x=w506, y=w505) -> (0:w504:bool)
                      }
                      frame #1 {
                        w509 = 16 ("contador eventos")
                        n360 = local write "TS_Ch_16"(w512) -> ()
                        n361 = local read "Veces canal"() -> (w507:u32[])
                        n362 = Index Array(array=w507, index=w509) -> (element=w510:u32)
                        n363 = Increment(x=w510) -> (x+1=w511:u32)
                        n364 = Replace Array Subset(array=w507, new element=w511, index=w509) -> (w508:u32[])
                        n365 = local write "Veces canal"(w508) -> ()
                      }
                    }
                  }
                  frame 17 {
                    n366 = flat-sequence {
                      tunnel: w515 -> [w517]
                      tunnel: [w516] -> w513
                      tunnel: w514 -> [w524]
                      frame #0 {
                        n367 = local read "TS_Ch_17"() -> (w518:u32)
                        n368 = Greater?(x=w518, y=w517) -> (0:w516:bool)
                      }
                      frame #1 {
                        w521 = 17 ("contador eventos")
                        n369 = local write "TS_Ch_17"(w524) -> ()
                        n370 = local read "Veces canal"() -> (w519:u32[])
                        n371 = Index Array(array=w519, index=w521) -> (element=w522:u32)
                        n372 = Increment(x=w522) -> (x+1=w523:u32)
                        n373 = Replace Array Subset(array=w519, new element=w523, index=w521) -> (w520:u32[])
                        n374 = local write "Veces canal"(w520) -> ()
                      }
                    }
                  }
                  frame 18 {
                    n375 = flat-sequence {
                      tunnel: w527 -> [w529]
                      tunnel: [w528] -> w525
                      tunnel: w526 -> [w536]
                      frame #0 {
                        n376 = local read "TS_Ch_18"() -> (w530:u32)
                        n377 = Greater?(x=w530, y=w529) -> (0:w528:bool)
                      }
                      frame #1 {
                        w533 = 18 ("contador eventos")
                        n378 = local write "TS_Ch_18"(w536) -> ()
                        n379 = local read "Veces canal"() -> (w531:u32[])
                        n380 = Index Array(array=w531, index=w533) -> (element=w534:u32)
                        n381 = Increment(x=w534) -> (x+1=w535:u32)
                        n382 = Replace Array Subset(array=w531, new element=w535, index=w533) -> (w532:u32[])
                        n383 = local write "Veces canal"(w532) -> ()
                      }
                    }
                  }
                  frame 19 {
                    n384 = flat-sequence {
                      tunnel: w539 -> [w541]
                      tunnel: [w540] -> w537
                      tunnel: w538 -> [w548]
                      frame #0 {
                        n385 = local read "TS_Ch 19"() -> (w542:u32)
                        n386 = Greater?(x=w542, y=w541) -> (0:w540:bool)
                      }
                      frame #1 {
                        w545 = 19 ("contador eventos")
                        n387 = local write "TS_Ch 19"(w548) -> ()
                        n388 = local read "Veces canal"() -> (w544:u32[])
                        n389 = Index Array(array=w544, index=w545) -> (element=w546:u32)
                        n390 = Increment(x=w546) -> (x+1=w547:u32)
                        n391 = Replace Array Subset(array=w544, new element=w547, index=w545) -> (w543:u32[])
                        n392 = local write "Veces canal"(w543) -> ()
                      }
                    }
                  }
                  frame 20 {
                    n393 = flat-sequence {
                      tunnel: w551 -> [w553]
                      tunnel: [w552] -> w549
                      tunnel: w550 -> [w560]
                      frame #0 {
                        n394 = local read "TS_Ch_20"() -> (w554:u32)
                        n395 = Greater?(x=w554, y=w553) -> (0:w552:bool)
                      }
                      frame #1 {
                        w557 = 20 ("contador eventos")
                        n396 = local write "TS_Ch_20"(w560) -> ()
                        n397 = local read "Veces canal"() -> (w556:u32[])
                        n398 = Index Array(array=w556, index=w557) -> (element=w558:u32)
                        n399 = Increment(x=w558) -> (x+1=w559:u32)
                        n400 = Replace Array Subset(array=w556, new element=w559, index=w557) -> (w555:u32[])
                        n401 = local write "Veces canal"(w555) -> ()
                      }
                    }
                  }
                  frame 21 {
                    n402 = flat-sequence {
                      tunnel: w563 -> [w565]
                      tunnel: [w564] -> w561
                      tunnel: w562 -> [w572]
                      frame #0 {
                        n403 = local read "TS_Ch_21"() -> (w566:u32)
                        n404 = Greater?(x=w566, y=w565) -> (0:w564:bool)
                      }
                      frame #1 {
                        w569 = 21 ("contador eventos")
                        n405 = local write "TS_Ch_21"(w572) -> ()
                        n406 = local read "Veces canal"() -> (w568:u32[])
                        n407 = Index Array(array=w568, index=w569) -> (element=w570:u32)
                        n408 = Increment(x=w570) -> (x+1=w571:u32)
                        n409 = Replace Array Subset(array=w568, new element=w571, index=w569) -> (w567:u32[])
                        n410 = local write "Veces canal"(w567) -> ()
                      }
                    }
                  }
                  frame 22 {
                    n411 = flat-sequence {
                      tunnel: w575 -> [w577]
                      tunnel: [w576] -> w573
                      tunnel: w574 -> [w584]
                      frame #0 {
                        n412 = local read "TS_Ch_22"() -> (w578:u32)
                        n413 = Greater?(x=w578, y=w577) -> (0:w576:bool)
                      }
                      frame #1 {
                        w581 = 22 ("contador eventos")
                        n414 = local read "Veces canal"() -> (w579:u32[])
                        n415 = local write "TS_Ch_22"(w584) -> ()
                        n416 = Index Array(array=w579, index=w581) -> (element=w582:u32)
                        n417 = Increment(x=w582) -> (x+1=w583:u32)
                        n418 = Replace Array Subset(array=w579, new element=w583, index=w581) -> (w580:u32[])
                        n419 = local write "Veces canal"(w580) -> ()
                      }
                    }
                  }
                  frame 23 {
                    n420 = flat-sequence {
                      tunnel: w587 -> [w589]
                      tunnel: [w588] -> w585
                      tunnel: w586 -> [w596]
                      frame #0 {
                        n421 = local read "TS_Ch_23"() -> (w590:u32)
                        n422 = Greater?(x=w590, y=w589) -> (0:w588:bool)
                      }
                      frame #1 {
                        w593 = 23 ("contador eventos")
                        n423 = local read "Veces canal"() -> (w591:u32[])
                        n424 = local write "TS_Ch_23"(w596) -> ()
                        n425 = Index Array(array=w591, index=w593) -> (element=w594:u32)
                        n426 = Increment(x=w594) -> (x+1=w595:u32)
                        n427 = Replace Array Subset(array=w591, new element=w595, index=w593) -> (w592:u32[])
                        n428 = local write "Veces canal"(w592) -> ()
                      }
                    }
                  }
                  frame 24 {
                    n429 = flat-sequence {
                      tunnel: w599 -> [w601]
                      tunnel: [w600] -> w597
                      tunnel: w598 -> [w608]
                      frame #0 {
                        n430 = local read "TS_Ch_24"() -> (w602:u32)
                        n431 = Greater?(x=w602, y=w601) -> (0:w600:bool)
                      }
                      frame #1 {
                        w605 = 24 ("contador eventos")
                        n432 = local write "TS_Ch_24"(w608) -> ()
                        n433 = local read "Veces canal"() -> (w603:u32[])
                        n434 = Index Array(array=w603, index=w605) -> (element=w606:u32)
                        n435 = Increment(x=w606) -> (x+1=w607:u32)
                        n436 = Replace Array Subset(array=w603, new element=w607, index=w605) -> (w604:u32[])
                        n437 = local write "Veces canal"(w604) -> ()
                      }
                    }
                  }
                  frame 25 {
                    n438 = flat-sequence {
                      tunnel: w611 -> [w613]
                      tunnel: [w612] -> w609
                      tunnel: w610 -> [w620]
                      frame #0 {
                        n439 = local read "TS_Ch 25"() -> (w614:u32)
                        n440 = Greater?(x=w614, y=w613) -> (0:w612:bool)
                      }
                      frame #1 {
                        w617 = 25 ("contador eventos")
                        n441 = local write "TS_Ch 25"(w620) -> ()
                        n442 = local read "Veces canal"() -> (w615:u32[])
                        n443 = Index Array(array=w615, index=w617) -> (element=w618:u32)
                        n444 = Increment(x=w618) -> (x+1=w619:u32)
                        n445 = Replace Array Subset(array=w615, new element=w619, index=w617) -> (w616:u32[])
                        n446 = local write "Veces canal"(w616) -> ()
                      }
                    }
                  }
                  frame 26 {
                    n447 = flat-sequence {
                      tunnel: w623 -> [w625]
                      tunnel: [w624] -> w621
                      tunnel: w622 -> [w632]
                      frame #0 {
                        n448 = local read "TS_Ch_26"() -> (w626:u32)
                        n449 = Greater?(x=w626, y=w625) -> (0:w624:bool)
                      }
                      frame #1 {
                        w629 = 26 ("contador eventos")
                        n450 = local write "TS_Ch_26"(w632) -> ()
                        n451 = local read "Veces canal"() -> (w627:u32[])
                        n452 = Index Array(array=w627, index=w629) -> (element=w630:u32)
                        n453 = Increment(x=w630) -> (x+1=w631:u32)
                        n454 = Replace Array Subset(array=w627, new element=w631, index=w629) -> (w628:u32[])
                        n455 = local write "Veces canal"(w628) -> ()
                      }
                    }
                  }
                  frame 27 {
                    n456 = flat-sequence {
                      tunnel: w635 -> [w637]
                      tunnel: [w636] -> w633
                      tunnel: w634 -> [w644]
                      frame #0 {
                        n457 = local read "TS_Ch_27"() -> (w638:u32)
                        n458 = Greater?(x=w638, y=w637) -> (0:w636:bool)
                      }
                      frame #1 {
                        w641 = 27 ("contador eventos")
                        n459 = local write "TS_Ch_27"(w644) -> ()
                        n460 = local read "Veces canal"() -> (w640:u32[])
                        n461 = Index Array(array=w640, index=w641) -> (element=w642:u32)
                        n462 = Increment(x=w642) -> (x+1=w643:u32)
                        n463 = Replace Array Subset(array=w640, new element=w643, index=w641) -> (w639:u32[])
                        n464 = local write "Veces canal"(w639) -> ()
                      }
                    }
                  }
                  frame 28 {
                    n465 = flat-sequence {
                      tunnel: w647 -> [w649]
                      tunnel: [w648] -> w645
                      tunnel: w646 -> [w656]
                      frame #0 {
                        n466 = local read "TS_Ch_28"() -> (w650:u32)
                        n467 = Greater?(x=w650, y=w649) -> (0:w648:bool)
                      }
                      frame #1 {
                        w653 = 28 ("contador eventos")
                        n468 = local read "Veces canal"() -> (w651:u32[])
                        n469 = local write "TS_Ch_28"(w656) -> ()
                        n470 = Index Array(array=w651, index=w653) -> (element=w654:u32)
                        n471 = Increment(x=w654) -> (x+1=w655:u32)
                        n472 = Replace Array Subset(array=w651, new element=w655, index=w653) -> (w652:u32[])
                        n473 = local write "Veces canal"(w652) -> ()
                      }
                    }
                  }
                  frame 29 {
                    n474 = flat-sequence {
                      tunnel: w659 -> [w661]
                      tunnel: [w660] -> w657
                      tunnel: w658 -> [w668]
                      frame #0 {
                        n475 = local read "TS_Ch_29"() -> (w662:u32)
                        n476 = Greater?(x=w662, y=w661) -> (0:w660:bool)
                      }
                      frame #1 {
                        w665 = 29 ("contador eventos")
                        n477 = local write "TS_Ch_29"(w668) -> ()
                        n478 = local read "Veces canal"() -> (w663:u32[])
                        n479 = Index Array(array=w663, index=w665) -> (element=w666:u32)
                        n480 = Increment(x=w666) -> (x+1=w667:u32)
                        n481 = Replace Array Subset(array=w663, new element=w667, index=w665) -> (w664:u32[])
                        n482 = local write "Veces canal"(w664) -> ()
                      }
                    }
                  }
                  frame 30 {
                    n483 = flat-sequence {
                      tunnel: [w673] -> w669
                      tunnel: w670 -> [w672]
                      tunnel: w671 -> [w680]
                      frame #0 {
                        n484 = local read "TS_Ch_30"() -> (w674:u32)
                        n485 = Greater?(x=w674, y=w672) -> (0:w673:bool)
                      }
                      frame #1 {
                        w677 = 30 ("contador eventos")
                        n486 = local read "Veces canal"() -> (w676:u32[])
                        n487 = local write "TS_Ch_30"(w680) -> ()
                        n488 = Index Array(array=w676, index=w677) -> (element=w678:u32)
                        n489 = Increment(x=w678) -> (x+1=w679:u32)
                        n490 = Replace Array Subset(array=w676, new element=w679, index=w677) -> (w675:u32[])
                        n491 = local write "Veces canal"(w675) -> ()
                      }
                    }
                  }
                }
                "error time order" <- w251
                n492 = stacked-sequence {
                  tunnel: w260 -> [_ w299]
                  frame #0 {
                    n493 = local read "suma ancho pulso"() -> (w298:u32)
                    n494 = local read "ToT"() -> (w297:u32)
                    n495 = Add(x=w298, y=w297) -> (x+y=w296:u32)
                    n496 = local write "suma ancho pulso"(w296) -> ()
                    n497 = local read "Num Event"() -> (w295:u32)
                    n498 = Divide(x=w296, y=w295) -> (x/y=→"media pulso":dbl)
                  }
                  frame #1 {
                    n499 = local read "media pulso"() -> (w308:dbl)
                    n500 = Subtract(x=w299, y=w308) -> (x-y=w307:dbl)
                    n501 = local read "suma desviacon"() -> (w305:dbl)
                    n502 = Square(x=w307) -> (x^2=w306:dbl)
                    n503 = Add(x=w306, y=w305) -> (x+y=w304:dbl)
                    n504 = local write "suma desviacon"(w304) -> ()
                    n505 = local read "Num Event"() -> (w303:u32)
                    n506 = Decrement(x=w303) -> (x-1=w302:u32)
                    n507 = Divide(x=w304, y=w302) -> (x/y=w301:dbl)
                    n508 = Square Root(x=w301) -> (sqrt(x)=w300:dbl)
                    n509 = local write "desviacion tipica ancho"(w300) -> ()
                  }
                }
                n510 = local read "Veces canal"() -> (w254:u32[])
                n511 = local read "Canal TDC"() -> (w259:u32[])
                n512 = call "Convert to Dynamic Data"("Array"=w259) -> ("Dynamic Data Type"=w258:dynamicdata)  [unwired: 3 in]
                n513 = call "Convert to Dynamic Data2"("Array"=w254) -> ("Dynamic Data Type"=w253:dynamicdata)  [unwired: 3 in]
                n514 = Merge Signals(w258, w253) -> (w257:dynamicdata)
                n515 = Or(x=w252, y=w271) -> (x .or. y?=w270:bool)
                n516 = call "Build Table"("Signals"=w257) -> ("Table"=→"Table":string[][])  [unwired: 9 in, 1 out]
                n517 = Or(x=w251, y=w270) -> (x .or. y?=w268:bool)
              }
              n518 = case shown="True" "Show channel table" {
                frame False {
                  n519 = property on="Table" class="Tbl (strict)"("Visible"=FALSE) -> ()  [unwired: 2 in, 2 out]
                }
                frame True {
                  n520 = property on="Table" class="Tbl (strict)"("Visible"=TRUE) -> ()  [unwired: 2 in, 2 out]
                }
              }
              n521 = case shown="True" "see tot" {
                frame False {
                  n522 = property on="ToT" class="WFGraph (strict)"("Visible"=FALSE) -> ()  [unwired: 2 in, 2 out]
                }
                frame True {
                  n523 = property on="ToT" class="WFGraph (strict)"("Visible"=TRUE) -> ()  [unwired: 2 in, 2 out]
                }
              }
              n524 = case shown="True" "see channel" {
                frame False {
                  n525 = property on="Events/TDC channel" class="WFGraph (strict)"("Visible"=FALSE) -> ()  [unwired: 2 in, 2 out]
                }
                frame True {
                  n526 = property on="Events/TDC channel" class="WFGraph (strict)"("Visible"=TRUE) -> ()  [unwired: 2 in, 2 out]
                }
              }
              n527 = case shown="False" "see supertime  ns" {
                frame False {
                  n528 = property on="supertime ns" class="WFGraph (strict)"("Visible"=FALSE) -> ()  [unwired: 2 in, 2 out]
                }
                frame True {
                  n529 = property on="supertime ns" class="WFGraph (strict)"("Visible"=TRUE) -> ()  [unwired: 2 in, 2 out]
                }
              }
              n530 = case shown="False" "see supertime sec" {
                frame False {
                  n531 = property on="Supertime sec" class="WFGraph (strict)"("Visible"=FALSE) -> ()  [unwired: 2 in, 2 out]
                }
                frame True {
                  n532 = property on="Supertime sec" class="WFGraph (strict)"("Visible"=TRUE) -> ()  [unwired: 2 in, 2 out]
                }
              }
              n533 = case shown="True" "show udp index" {
                frame False {
                  n534 = property on="UDP INDEX" class="WFGraph (strict)"("Visible"=FALSE) -> ()  [unwired: 2 in, 2 out]
                }
                frame True {
                  n535 = property on="UDP INDEX" class="WFGraph (strict)"("Visible"=TRUE) -> ()  [unwired: 2 in, 2 out]
                }
              }
              n536 = case shown="False" "show event/index" {
                frame False {
                  n537 = property on="EVENT/index" class="WFGraph (strict)"("Visible"=FALSE) -> ()  [unwired: 2 in, 2 out]
                }
                frame True {
                  n538 = property on="EVENT/index" class="WFGraph (strict)"("Visible"=TRUE) -> ()  [unwired: 2 in, 2 out]
                }
              }
            }
          }
          n539 = Unbundle By Name(w47) -> ("status"=w43:bool)
          n540 = Or(x=w43, y="stop") -> (x .or. y?=w51:bool)
          n541 = Or(x=w51, y=w42) -> (x .or. y?=w52:bool)
          n542 = Or(x=w52, y=FALSE) -> (x .or. y?=w49:bool)
          "iteracion" <- w46
        }
      }
    }
    n543 = Or(x=w20, y=FALSE) -> (x .or. y?=w19:bool)
    n544 = Or(x=w19, y=w18) -> (x .or. y?=w17:bool)
  }
  n545 = local write "Show channel table"(w1) -> ()
  n546 = local write "see tot"(w1) -> ()
  n547 = local write "Arrival Time"(0) -> ()
  n548 = local write "Event Hex"("0") -> ()
  n549 = local write "see channel"(w1) -> ()
  n550 = local write "see supertime  ns"(w1) -> ()
  n551 = local write "show udp index"(w1) -> ()
  n552 = local write "see supertime sec"(w1) -> ()
  n553 = local write "show event/index"(w1) -> ()
  "Port" <- u16 56015
